vi "Main.vi"(8 "Error In":errorcluster) -> (0 "Error Out":errorcluster)   [LabVIEW 2018, in "ErrorHandler.lvlib"]
uses:
  ErrorHandler.lvlib
  InternalData.ctl
  UserEvents/StopUE.lvlib
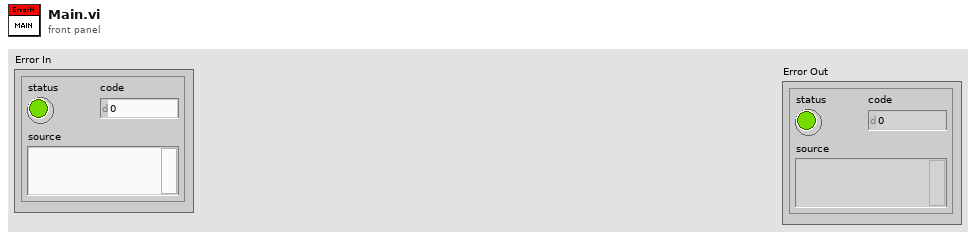
[diagram p1: front panel]
types:
  T1 = typedef "ErrorHandler.lvlib/InternalData.ctl" = cluster{"Status":string}
  T2 = typedef "ErrorHandler.lvlib/States_Module.ctl" = enum16{"Error", "DoSomething", "Shutdown", "Initialize"}
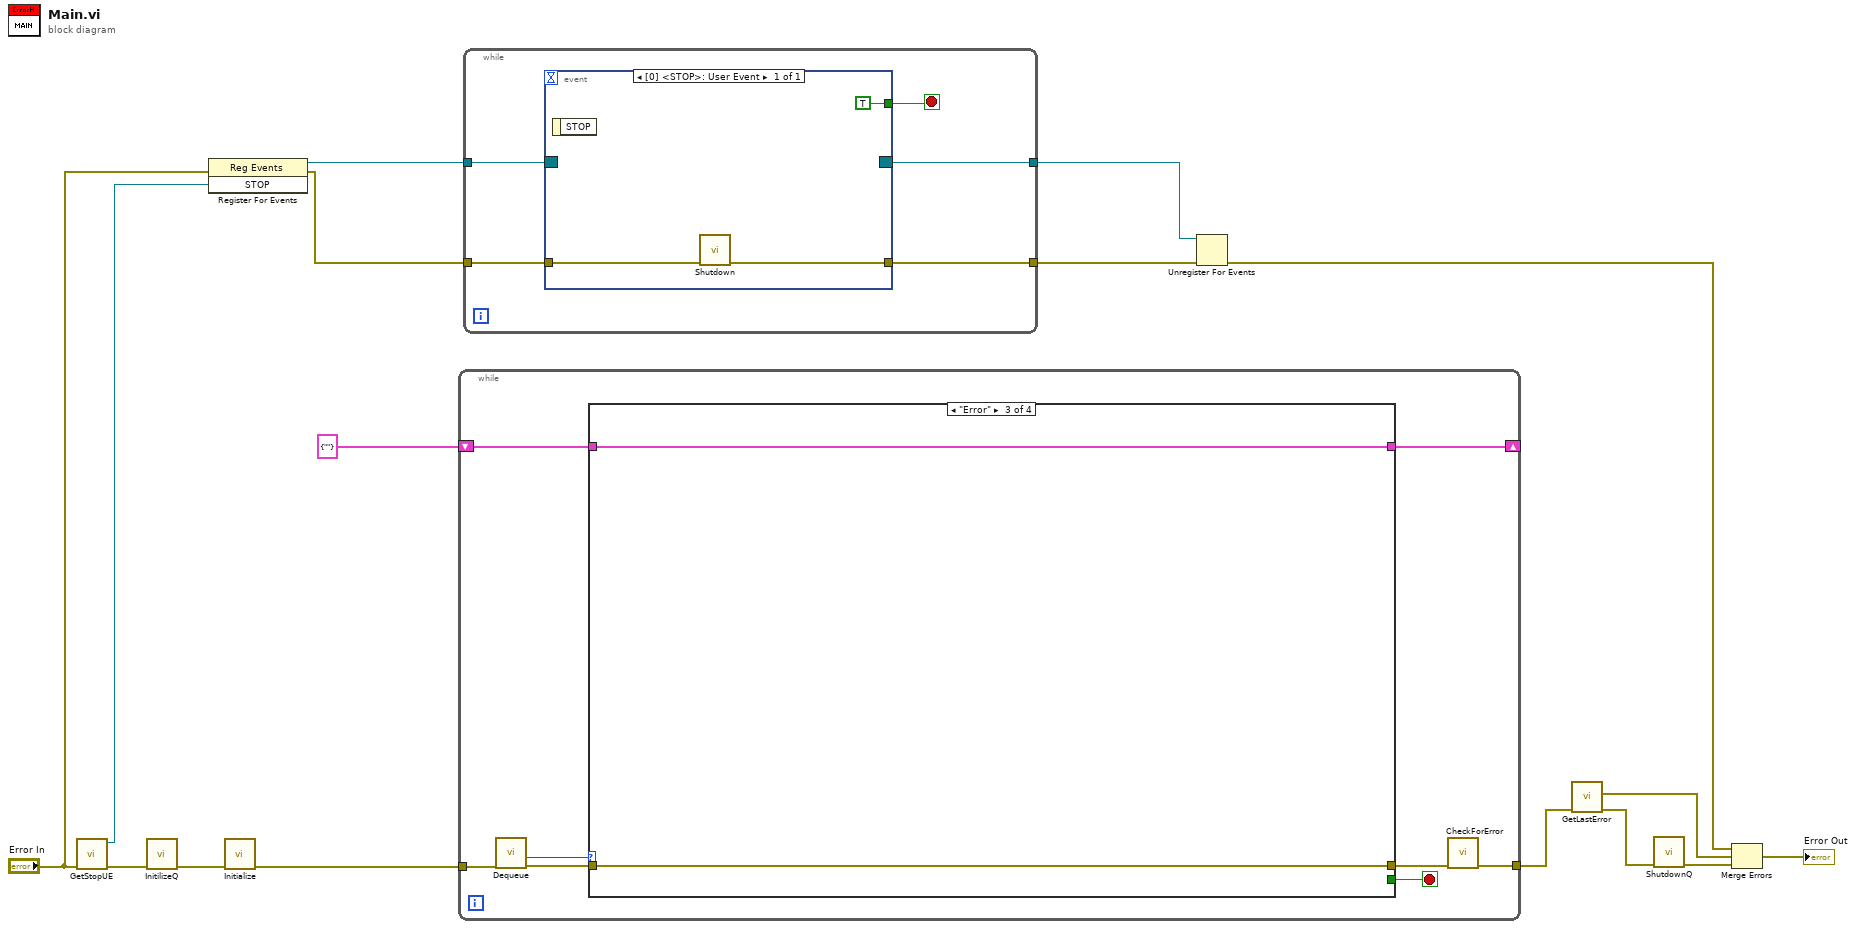
[diagram p0: block diagram]
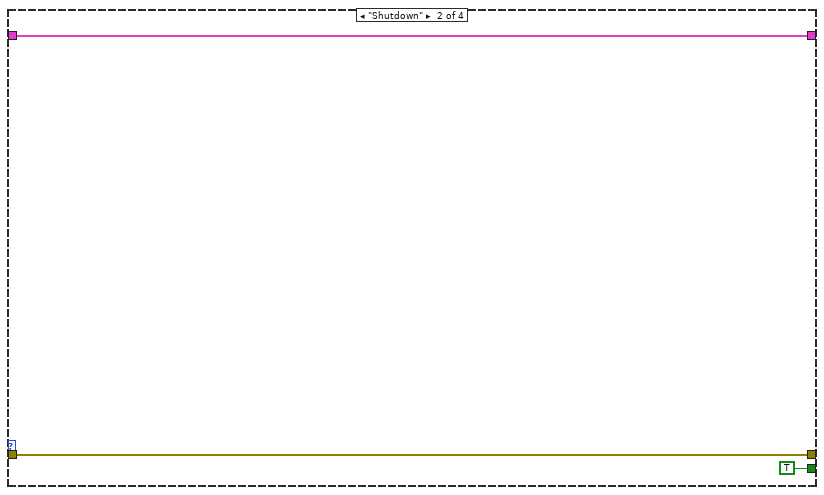
[diagram p3: hidden frame]
diagram:
  n1 = call "GetStopUE.vi"("Error In"="Error In") -> ("Error Out"=w13:errorcluster, "STOP"=w16:refnum<user-event>)  [unwired: 9 in]
  n2 = call "InitilizeQ.vi"("Error In"=w13) -> ("Error Out"=w11:errorcluster)  [unwired: 10 in]
  n3 = register-events(error in="Error In", w16) -> (reference out=w15:refnum<event-registration>, error out=w14:errorcluster)  [unwired: 1 in]
  n4 = call "Initialize.vi"("Error In"=w11) -> ("error out"=w10:errorcluster)  [unwired: 9 in, 1 out]
  n5 = while {
    tunnel: w10 -> [w24]
    tunnel: [w17] -> w7
    shift-right: [w19] -> _
    shift-left: T1 {"Status"=""} ("InternalData") -> [w20]
    stop <- w21 stop-if-true
    n6 = call "Dequeue.vi"("Error In"=w24) -> ("error out"=w23:errorcluster, "State"=w22:T2)  [unwired: 8 in, 1 out]
    n7 = case shown="\"Error\"" w22 {
      tunnel: w23 -> [w26 w28 w31 w33]
      tunnel: [_ TRUE _ _] -> w21
      tunnel: [w26 w28 w31 w33] -> w18
      tunnel: w20 -> [w25 w27 w30 w32]
      tunnel: [w25 w27 w30 w32] -> w19
      frame "DoSomething", Default {
      }
      frame "Shutdown" {
      }
      frame "Error" {
      }
      frame "Initialize" {
      }
    }
    n8 = call "CheckForError.vi"("Error In"=w18) -> ("error out"=w17:errorcluster)  [unwired: 10 in]
  }
  n9 = while {
    tunnel: w15 -> [w38]
    tunnel: w14 -> [w36]
    tunnel: [w35] -> w9
    tunnel: [w34] -> w8
    stop <- w37 stop-if-true
    n10 = event shown="[0] <STOP>: User Event" {
      selector: w38 -> [_]
      dyn-events: [_] -> w34
      timeout: _ -> [_]
      tunnel: [TRUE] -> w37
      tunnel: w36 -> [w40]
      tunnel: [w39] -> w35
      event User Event {
        n11 = event-data() -> ()  [unwired: 1 in, 1 out]
        n12 = call "Shutdown.vi"("Error In"=w40) -> ("error out"=w39:errorcluster)  [unwired: 9 in, 1 out]
      }
    }
  }
  n13 = Unregister For Events(event registration refnum=w8, error in=w9) -> (error out=w3:errorcluster)
  n14 = call "GetLastError.vi"("Error In"=w7) -> ("error IO"=w6:errorcluster, "Last Error"=w4:errorcluster)  [unwired: 9 in]
  n15 = call "ShutdownQ.vi"("Error In"=w6) -> ("Error Out"=w5:errorcluster)  [unwired: 10 in]
  n16 = Merge Errors(w3, w4, w5) -> (→"Error Out":errorcluster)
